vi "Drag Edge Point.vi"(0 "FSM.Graph In":refnum<class "FSM.Graph.lvclass">, 5 "Location":cluster{"x":i16, "y":i16}) -> (4 "FSM.Graph Out":refnum<class "FSM.Graph.lvclass">)   [LabVIEW 2020, in "FSM.Graph.lvclass"]
uses:
  FSM.Graph.lvclass
  FSM.Graph.lvclass/FSM.Graph.ctl
  FSM.Edge/FSM.Edge.lvclass
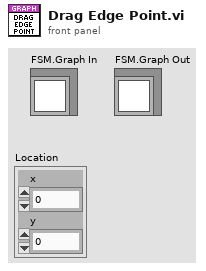
[diagram p1: front panel]
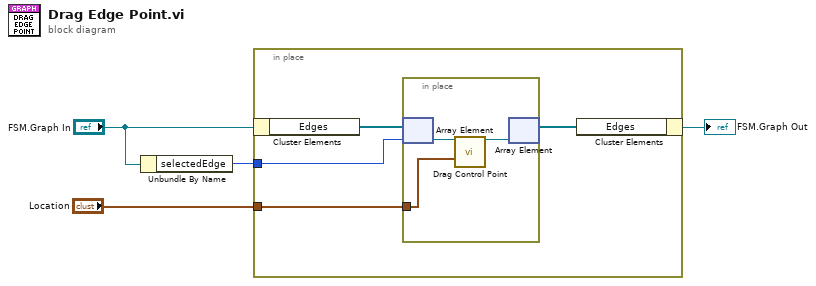
[diagram p0: block diagram]
diagram:
  n1 = Unbundle By Name("FSM.Graph In") -> ("selectedEdge"=w3:i32)
  n2 = in-place {
    in-place-border: w3 -> [w7]
    in-place-border: "Location" -> [w6]
    n3 = in-place-cluster #1("FSM.Graph In") -> ("Edges"=w8:refnum<class "FSM.Edge.lvclass">[])
    n4 = in-place {
      in-place-border: w6 -> [w10]
      n5 = in-place-array #2(w8, w7) -> (w11:refnum<class "FSM.Edge.lvclass">)
      n6 = call "Drag Control Point.vi"("FSM.Edge In"=w11, "location"=w10) -> ("FSM.Edge Out"=w9:refnum<class "FSM.Edge.lvclass">)  [unwired: 13 in]
      n7 = in-place-array #2(w9) -> (w5:refnum<class "FSM.Edge.lvclass">[])  [unwired: 1 out]
    }
    n8 = in-place-cluster #1("Edges"=w5) -> (→"FSM.Graph Out":refnum<class "FSM.Graph.lvclass">)
  }
